vi "acquisitionDisplayVolume.vi"(1 "z":dbl[](array[numeric]), 2 "frames":u16[][][](array[numeric])) -> ()   [LabVIEW 2017]
panel:
  in  "adjust y scale (to area)":bool
  out "Delta z":dbl
  in  "adjust y scale (to cursors)":bool
  out "single frame":T1(plugin-control)
  out "z profile of area":cluster{"X":dbl, "Y":dbl}[](graph)
  in  "deltaY":i32=4
  in  "deltaX":i32=8
  in  "Y0":i32=544
  in  "X0":i32=216
  out "single frame":u16[][](graph)
  in  "plane index":i32
  out "axis-summed frame":u64[][](graph)
  in  "axis":u16(ring)=2 items=["x", "y", "z"]
  in  "stop":bool
  # "USE THIS VI TO DISPLAY A VOLUME"
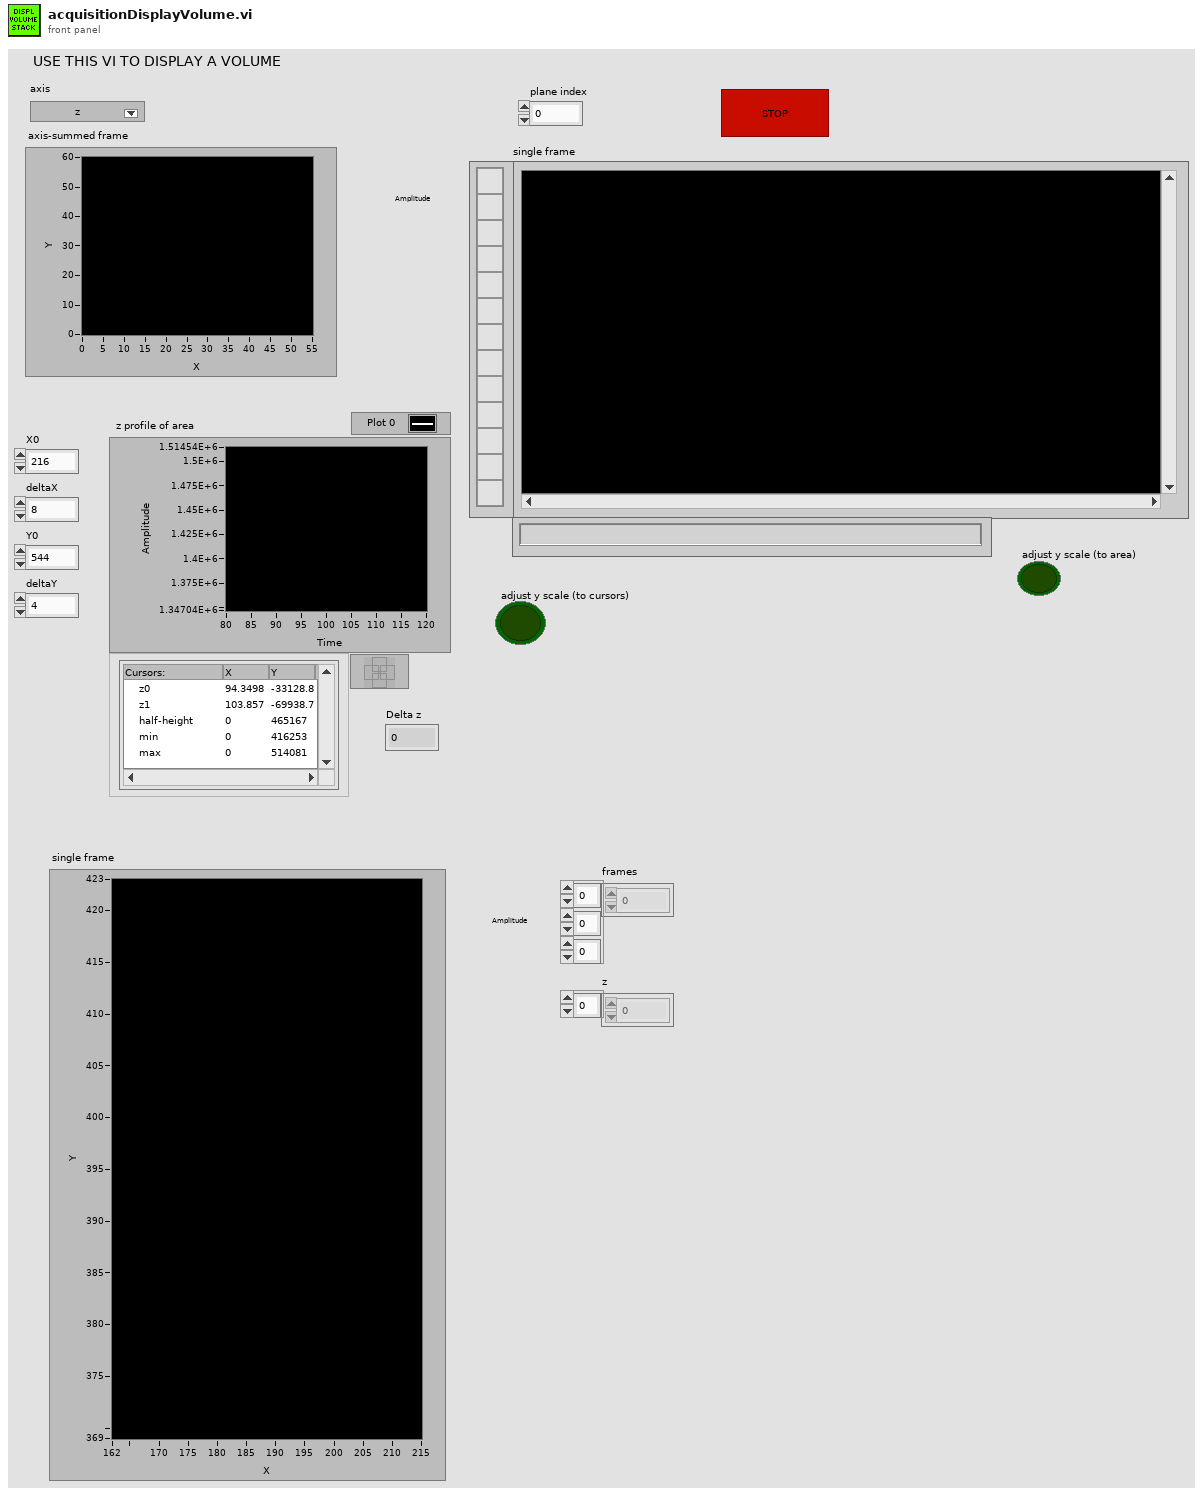
[diagram p1: front panel]
types:
  T1 = typedef "IMAQ Image.ctl" = refnum<image>
  T2 = typedef "Image Type" = u32
  T3 = typedef "LVCursorListTypeDef.ctl" = cluster{"Name":string, "Color":u32, "Style":u8, "Point Style":u8, "Name Visible":bool, "Allow Drag":bool, "Cursor Mode":u32, "Plot":i32, "Index":i32, "Position":cluster{"X":dbl, "Y":dbl}, "X Scale":u32, "Y Scale":u32, "Watch Plots":i32[], "Watch All Plots":bool, "Plot Area":i32, "Label Offset":cluster{"X":dbl, "Y":dbl}}[]
  T4 = cluster{"Global Rectangle":i32[], "Contours":cluster{"Contour Type":u32, "ROI Type":u32, "Points":i32[]}[]}
  T5 = typedef "IMAQ Rectangle" = cluster{"Left":i32, "Top":i32, "Right":i32, "Bottom":i32, "Rotation":dbl}
  T6 = cluster{"Name":string, "Color":u32, "Style":u8, "Point Style":u8, "Name Visible":bool, "Allow Drag":bool, "Cursor Mode":u32, "Plot":i32, "Index":i32, "Position":cluster{"X":dbl, "Y":dbl}, "X Scale":u32, "Y Scale":u32, "Watch Plots":i32[], "Watch All Plots":bool, "Plot Area":i32, "Label Offset":cluster{"X":dbl, "Y":dbl}}
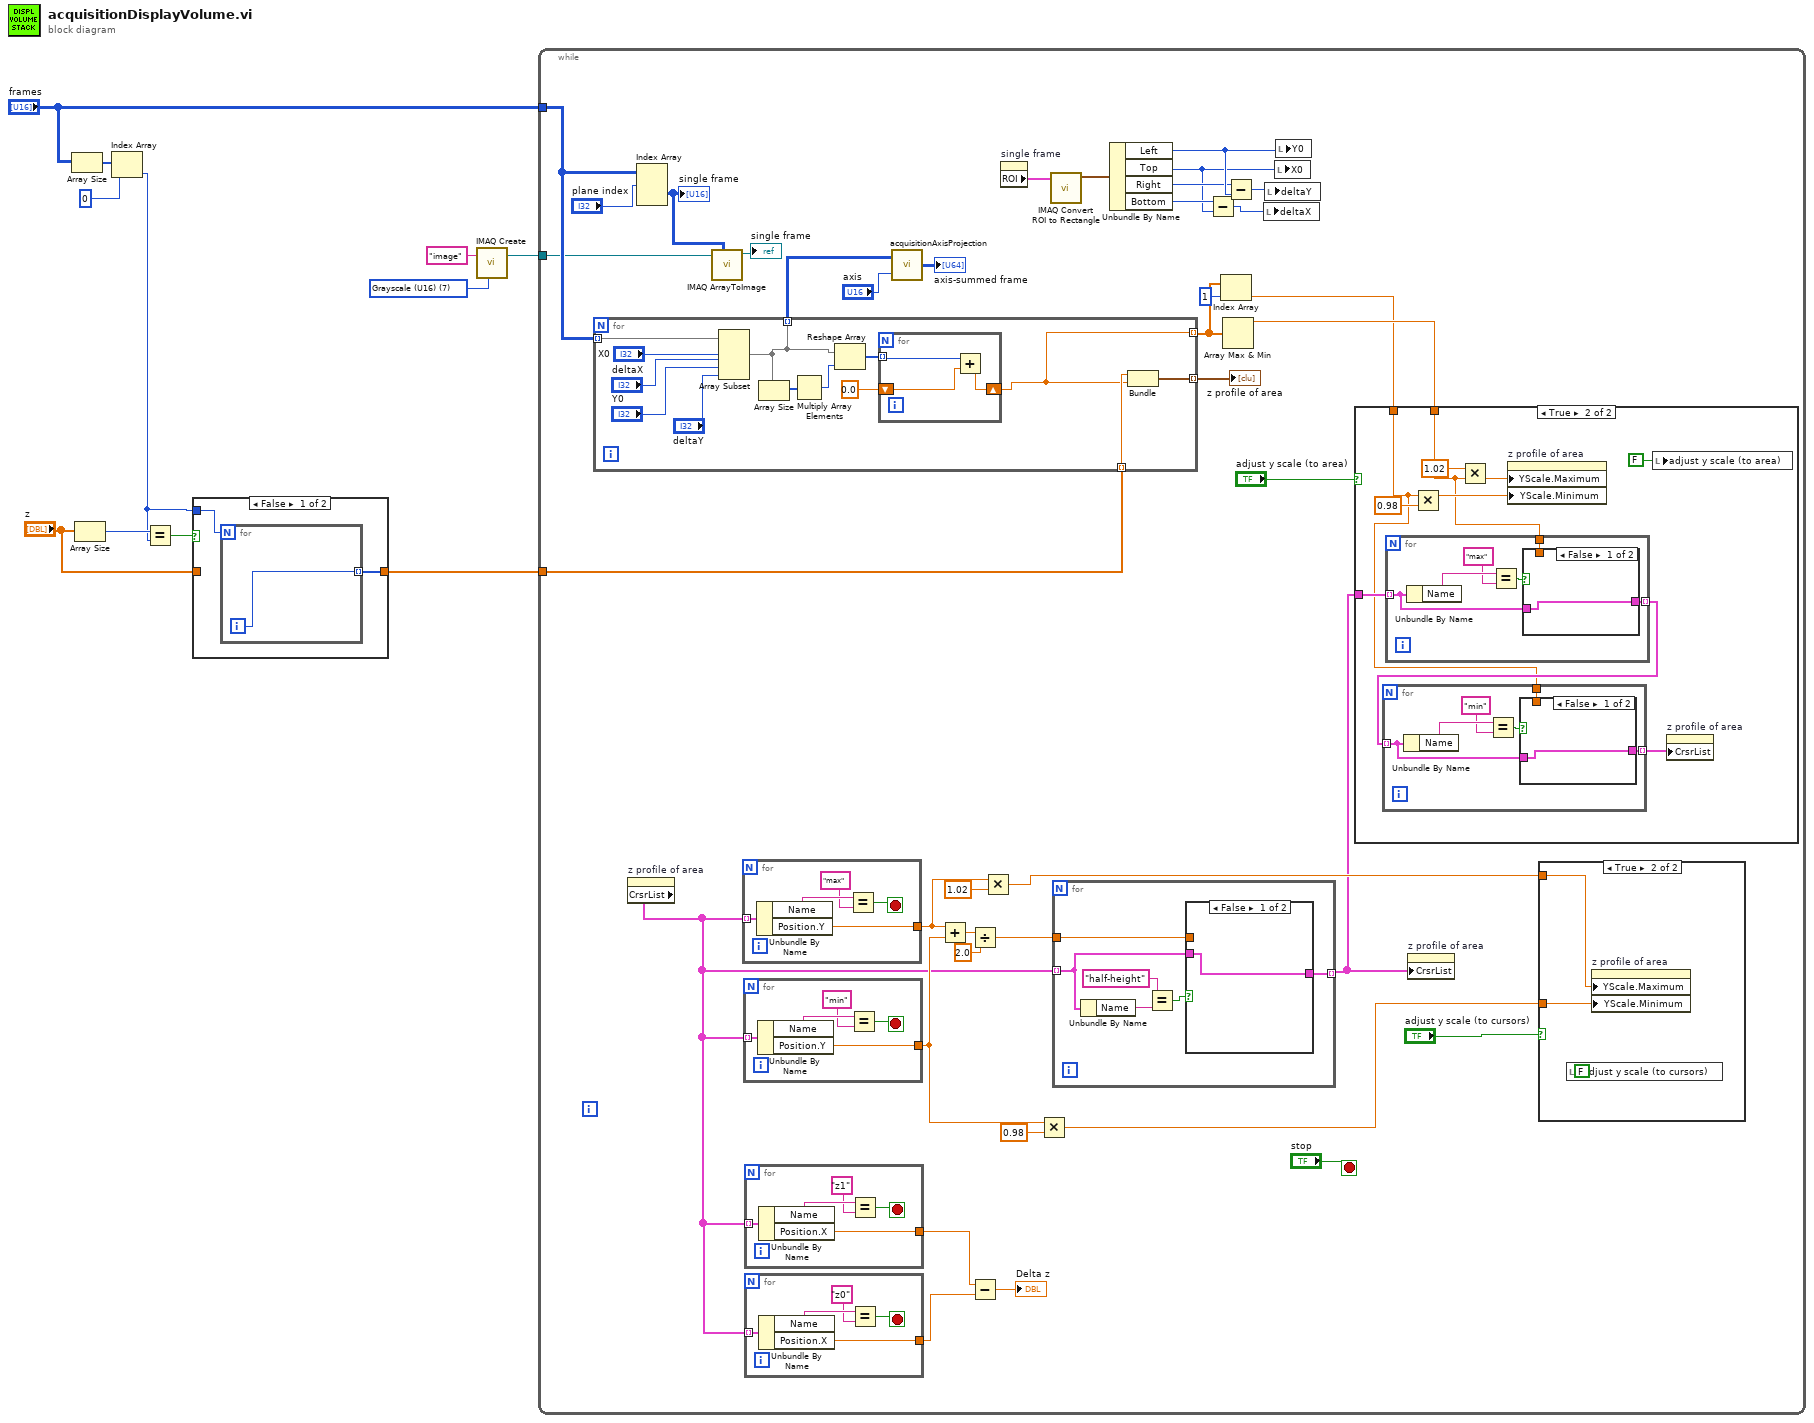
[diagram p0: block diagram]
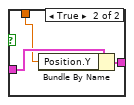
[diagram p4: hidden frame]
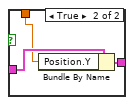
[diagram p5: hidden frame]
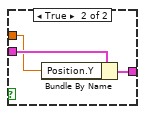
[diagram p7: hidden frame]
diagram:
  w1 = T2 7 items=["Grayscale (U8)", "Grayscale (I16)", "Grayscale (SGL)", "Complex (CSG)", "RGB (U32)", "HSL (U32)", "RGB (U64)", "Grayscale (U16)"] ("Image Type")
  n1 = Array Size(array="frames") -> (size(s)=w10:i32[])
  n2 = Array Size(array="z") -> (size(s)=w8:i32)
  n3 = Index Array(array=w10, index=0) -> (element=w4:i32)
  n4 = Equal?(x=w8, y=w4) -> (x = y?=w7:bool)
  n5 = case shown="False" w7 {
    tunnel: [w12 w15] -> w5
    tunnel: "z" -> [_ w15]
    tunnel: w4 -> [w13 _]
    frame False {
      n6 = for {
        N: w13 -> [_]
        tunnel: [w14] -> w12 mode=indexing
        i -> [w14]
      }
    }
    frame True {
    }
  }
  n7 = call "IMAQ Create"("Image Name"="image", "Image Type"=w1) -> ("New Image"=w3:T1)  [unwired: 3 in, 1 out]
  n8 = while {
    tunnel: "frames" -> [w50]
    tunnel: w5 -> [w49]
    tunnel: w3 -> [w47]
    stop <- "stop" stop-if-true
    n9 = for {
      tunnel: w50 -> [w130] mode=indexing
      tunnel: w49 -> [w121] mode=indexing
      tunnel: [w120] -> w48 mode=indexing
      tunnel: [w119] -> w36 mode=indexing
      tunnel: [w118] -> w20 mode=indexing
      n10 = Array Subset(array=w130, index (row)="X0", length (row)="deltaX", index (col)="Y0", length (col)="deltaY") -> (w119:u16[][])
      n11 = Array Size(array=w119) -> (size(s)=w124:i32[])
      n12 = Multiply Array Elements(1:w124) -> (0:w125:i32)
      n13 = Reshape Array(w119, w125) -> (w123:u16[])
      n14 = for {
        tunnel: w123 -> [w133] mode=indexing
        shift-right: [w131] -> w118
        shift-left: 0.0 -> [w132]
        n15 = Add(x=w133, y=w132) -> (x+y=w131:dbl)
      }
      n16 = Bundle("Numeric"=w121, w118) -> (w120:cluster{"Numeric":dbl, dbl})  [unwired: 1 in]
    }
    "z profile of area" <- w48
    n17 = property on="z profile of area" class="XYGraph (strict)"() -> ("CrsrList"=w17:T3)  [unwired: 2 in, 2 out]
    n18 = Index Array(array=w50, index (dim 0)="plane index") -> (element=w46:u16[][])  [unwired: 2 in]
    "single frame" <- w46
    n19 = call "IMAQ ArrayToImage"("Image Pixels (U16)"=w46, "Image"=w47) -> ("Image Out"=→"single frame":T1)  [unwired: 8 in, 1 out]
    n20 = for {
      tunnel: w17 -> [w117] mode=indexing
      tunnel: [w113] -> w30
      stop <- w114 stop-if-true
      n21 = Unbundle By Name(w117) -> ("Name"=w116:string, "Position.Y"=w113:dbl)
      n22 = Equal?(x=w116, y="max") -> (x = y?=w114:bool)
    }
    n23 = for {
      tunnel: w17 -> [w112] mode=indexing
      tunnel: [w108] -> w32
      stop <- w109 stop-if-true
      n24 = Unbundle By Name(w112) -> ("Name"=w111:string, "Position.Y"=w108:dbl)
      n25 = Equal?(x=w111, y="min") -> (x = y?=w109:bool)
    }
    n26 = for {
      tunnel: w17 -> [w94] mode=indexing
      tunnel: [w90] -> w25
      stop <- w91 stop-if-true
      n27 = Unbundle By Name(w94) -> ("Name"=w93:string, "Position.X"=w90:dbl)
      n28 = Equal?(x=w93, y="z1") -> (x = y?=w91:bool)
    }
    n29 = for {
      tunnel: w17 -> [w89] mode=indexing
      tunnel: [w85] -> w24
      stop <- w86 stop-if-true
      n30 = Unbundle By Name(w89) -> ("Name"=w88:string, "Position.X"=w85:dbl)
      n31 = Equal?(x=w88, y="z0") -> (x = y?=w86:bool)
    }
    n32 = call "acquisitionAxisProjection.vi"("axis (z)"="axis", "z stack"=w36) -> ("projected img"=→"axis-summed frame":u64[][])
    n33 = Add(x=w30, y=w32) -> (x+y=w35:dbl)
    n34 = Divide(x=w35, y=2.0) -> (x/y=w33:dbl)
    n35 = Subtract(x=w25, y=w24) -> (x-y=→"Delta z":dbl)
    n36 = Multiply(x=w30, y=1.02) -> (x*y=w27:dbl)
    n37 = property on="single frame" class="ImageControl"() -> ("ROI"=w44:T4)  [unwired: 2 in, 2 out]
    n38 = Multiply(x=w32, y=0.98) -> (x*y=w26:dbl)
    n39 = call "IMAQ Convert ROI to Rectangle"("ROI Descriptor"=w44) -> ("Rectangle"=w43:T5)  [unwired: 8 in, 1 out]
    n40 = for {
      tunnel: w17 -> [w99] mode=indexing
      tunnel: w33 -> [w100]
      tunnel: [w98] -> w16 mode=indexing
      n41 = Unbundle By Name(w99) -> ("Name"=w103:string)
      n42 = Equal?(x="half-height" ("y"), y=w103) -> (x = y?=w101:bool)
      n43 = case shown="False" w101 {
        tunnel: w100 -> [_ w106]
        tunnel: w99 -> [w104 w107]
        tunnel: [w104 w105] -> w98
        frame False {
        }
        frame True {
          n44 = Bundle By Name(cluster=w107, "Position.Y"=w106) -> (w105:T6)
        }
      }
    }
    n45 = Unbundle By Name(w43) -> ("Left"=w42:i32, "Top"=w37:i32, "Right"=w39:i32, "Bottom"=w40:i32)
    n46 = Subtract(x=w40, y=w37) -> (x-y=w38:i32)
    n47 = Index Array(array=w20, index=1) -> (element=w18:dbl)
    n48 = Array Max & Min(array=w20) -> (max value=w21:dbl)  [unwired: 3 out]
    n49 = Subtract(x=w39, y=w42) -> (x-y=w41:i32)
    n50 = local write "deltaX"(w38) -> ()
    n51 = local write "deltaY"(w41) -> ()
    n52 = local write "X0"(w37) -> ()
    n53 = local write "Y0"(w42) -> ()
    n54 = case shown="True" "adjust y scale (to area)" {
      tunnel: w21 -> [_ w59]
      tunnel: w18 -> [_ w57]
      tunnel: w16 -> [_ w60]
      frame False {
      }
      frame True {
        n55 = for {
          tunnel: w60 -> [w76] mode=indexing
          tunnel: w59 -> [w77]
          tunnel: [w75] -> w58 mode=indexing
          n56 = Unbundle By Name(w76) -> ("Name"=w80:string)
          n57 = Equal?(x=w80, y="max") -> (x = y?=w78:bool)
          n58 = case shown="False" w78 {
            tunnel: w77 -> [_ w83]
            tunnel: w76 -> [w81 w84]
            tunnel: [w81 w82] -> w75
            frame False {
            }
            frame True {
              n59 = Bundle By Name(cluster=w84, "Position.Y"=w83) -> (w82:T6)
            }
          }
        }
        n60 = for {
          tunnel: w58 -> [w66] mode=indexing
          tunnel: w57 -> [w67]
          tunnel: [w65] -> w56 mode=indexing
          n61 = Unbundle By Name(w66) -> ("Name"=w70:string)
          n62 = Equal?(x=w70, y="min") -> (x = y?=w68:bool)
          n63 = case shown="False" w68 {
            tunnel: w67 -> [_ w73]
            tunnel: w66 -> [w71 w74]
            tunnel: [w71 w72] -> w65
            frame False {
            }
            frame True {
              n64 = Bundle By Name(cluster=w74, "Position.Y"=w73) -> (w72:T6)
            }
          }
        }
        n65 = Multiply(x=w57, y=0.98) -> (x*y=w64:dbl)
        n66 = Multiply(x=1.02, y=w59) -> (x*y=w62:dbl)
        n67 = property on="z profile of area" class="XYGraph (strict)"("YScale.Maximum"=w62, "YScale.Minimum"=w64) -> ()  [unwired: 2 in, 2 out]
        n68 = local write "adjust y scale (to area)"(FALSE ("adjust y scale (to area)")) -> ()
        n69 = property on="z profile of area" class="XYGraph (strict)"("CrsrList"=w56) -> ()  [unwired: 2 in, 2 out]
      }
    }
    n70 = property on="z profile of area" class="XYGraph (strict)"("CrsrList"=w16) -> ()  [unwired: 2 in, 2 out]
    n71 = case shown="True" "adjust y scale (to cursors)" {
      tunnel: w27 -> [_ w97]
      tunnel: w26 -> [_ w96]
      frame False {
      }
      frame True {
        n72 = local write "adjust y scale (to cursors)"(FALSE ("adjust z scale")) -> ()
        n73 = property on="z profile of area" class="XYGraph (strict)"("YScale.Maximum"=w97, "YScale.Minimum"=w96) -> ()  [unwired: 2 in, 2 out]
      }
    }
  }
